vi "Begin.vi"(8 "error in":errorcluster) -> (0 "error out":errorcluster)   [LabVIEW 2016]
doc: "Called before other user functions, this VI is expected to open initial I/O refnums, load in file data, and do all program initialization. Notice that the <B>error out</B> terminal is simply used for data flow. Wiring it to other structures or subVIs ensures that this VI runs first."
uses:
  <vilib>/Rock Robotics/WPI/Solenoid/WPI_SolenoidValue.ctl
  <vilib>/Rock Robotics/WPI/ThirdParty/CanMotor/TalonSRX/WPI_CANTalonSRX_APIControlMode.ctl
  <vilib>/Rock Robotics/WPI/ThirdParty/CanMotor/TalonSRX/WPI_CANTalonSRX_BrakeOverride.ctl
  <vilib>/Rock Robotics/WPI/ThirdParty/CanMotor/TalonSRX/WPI_CANTalonSRX_APIFeedbackSelect.ctl
  <vilib>/Rock Robotics/WPI/SafetyOutput/WPI_SafetyOutputConfigMenu.ctl
  Constants/Private/Private Global.vi
  <vilib>/Rock Robotics/WPI/Solenoid/WPI_SolenoidOpenDouble.vi
  <vilib>/Rock Robotics/WPI/RobotDrive/WPI_RobotDriveOpen2MotorWithSPARK.vi
  <vilib>/Rock Robotics/WPI/MotorControl/WPI_MotorControlOpen SPARK.vi
  <vilib>/Rock Robotics/WPI/Counter/WPI_CounterDigitalInputToDigitalSource.vi
  <vilib>/Rock Robotics/Network Tables/NT Write String Array.vi
  <vilib>/Rock Robotics/WPI/Solenoid/WPI_SolenoidSetEnum.vi
  Constants/Constants.lvlib
  SubSystems/Path Track/Path Track.lvlib
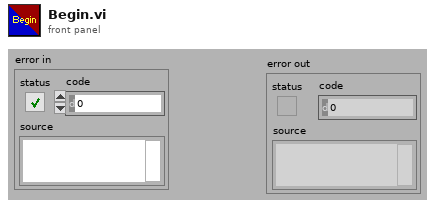
[diagram p1: front panel]
types:
  T1 = typedef "WPI_SafetyOutputConfigMenu.ctl" = enum16{"Enable", "Disable"}
  T2 = typedef "WPI_CANTalonSRX_APIControlMode.ctl" = enum8{"Percent VBus", "Speed", "Position", "Slave", "Unchanged / Invalid", "Voltage Compensation", "Current", "Motion Profile", "Motion Magic"}
  T3 = typedef "WPI_CANTalonSRX_APIFeedbackSelect.ctl" = enum16{"Digital Quadrature Encoder", "Analog Potentiometer", "Analog Encoder", "Count on Quad-A (Rising-Edge)", "Count on Quad-A (Falling-Edge)", "CTR Magnetic Enc (Absolute)", "CTR Magnetic Enc (Relative)", "Pulse Width"}
  T4 = typedef "WPI_CANTalonSRX_BrakeOverride.ctl" = enum8{"No Override", "Override to Coast", "Override to Brake"}
  T5 = typedef "WPI_SolenoidValue.ctl" = enum16{"Off", "On", "Forward", "Reverse"}
  T6 = typedef "Constants.lvlib/Constants.ctl" = cluster{"Port Layout":cluster{"RightMotorInverted":bool, "LeftMotorInverted":bool, "Left Motors":T7, "Right Motors":T7, "Auton List":string[], "XBOX Port":T8, "Encoder L A":T9, "Encoder L B":T9, "Encoder R A":T9, "Encoder R B":T9, "L Encoder Inverse":bool, "R Encoder Inverse":bool, "Drive Distance per Count":dbl, "Gyro Bus":T10, "Fuel Roller 1":T7, "Front Roller":T7, "Gear Flipper":T7, "Climber 1":T7, "Fuel Roller Invert":bool, "Front Roller Invert":bool, "Gear Flipper Invert":bool, "Climber Invert":bool, "PCM":u8, "Fuel Roller 2":T7, "Gear Sensor":T11, "Gear Release Fwd":T12, "Gear Release Rvrs":T12, "Fuel Arm Fwd":T12, "Fuel Arm Rvrs":T12, "Shifter Fwrd":T12, "Shifter Rvrs":T12, "Climber 2":T7, "PDP":u8, "Shooter Front Channel":u8, "Shooter Rear Channel":u8, "Shooter Feed Channel":u8, "Camera Servo":T7, "Gear Servo":T7, "Gear Puncher Fwrd":T12, "Gear Puncher Rvrs":T12, "Shooter Inverse":bool, "Ring Light Switch":T9}, "Drive Constants":cluster{"Wheelbase In.":dbl, "Max Velocity (In/sec)":dbl, "Max Accel (In/sec^2)":dbl, "Max Jerk (In/sec^3)":dbl, "Path dt":dbl, "Path Sample Count":i32, "Deadband":dbl}, "Arm System":cluster{"Front Roller Gear Speed":dbl, "Front Roller Fuel Speed":dbl, "Gear Flipper Speed":dbl, "Fuel Roller Speed":dbl, "Gear Release Wait (ms)":i32, "Gear Sensor Threshold":dbl, "Flappy Open Angle":i32, "Flappy Close Angle":i32, "Ramp Rate (EGU/min)":dbl}, "Shooter":cluster{"Shooter Wheels":cluster{"P":dbl, "I":dbl, "D":dbl, "F":dbl, "IZone":dbl}, "Feeder":cluster{"P":dbl, "I":dbl, "D":dbl, "F":dbl, "IZone":dbl}, "Front Shooter RPM":dbl, "Rear Shooter RPM":dbl, "Agitator Speed":dbl, "Feeder Speed":dbl, "Shooter CPR":u32, "Feeder CPR":u32}, "Vision":cluster{"High Goal Height (in.)":dbl, "Low Goal Height (in.)":dbl, "Camera Height High (in.)":dbl, "Camera Height Low (in.)":dbl, "Servo Pitch Gear (deg)":dbl, "Camera Yaw (deg)":dbl, "Servo Gear":i32, "Servo Boiler":i32, "Servo Pitch Boiler (deg)":dbl}}
  T7 = typedef "FPGA_DIOPWMChannel.ctl" = enum8{"PWM 0", "PWM 1", "PWM 2", "PWM 3", "PWM 4", "PWM 5", "PWM 6", "PWM 7", "PWM 8", "PWM 9", "PWM MXP 0", "PWM MXP 1", "PWM MXP 2", "PWM MXP 3", "PWM MXP 4", "PWM MXP 5", "PWM MXP 6", "PWM MXP 7", "PWM MXP 8", "PWM MXP 9", "Invalid"}
  T8 = typedef "WPI_JoystickDeviceEnum.ctl" = enum16{"USB 0", "USB 1", "USB 2", "USB 3", "USB 4", "USB 5"}
  T9 = typedef "FPGA_DIOChannel.ctl" = enum8{"DIO 0", "DIO 1", "DIO 2", "DIO 3", "DIO 4", "DIO 5", "DIO 6", "DIO 7", "DIO 8", "DIO 9", "DIO MXP 0", "DIO MXP 1", "DIO MXP 2", "DIO MXP 3", "DIO MXP 4", "DIO MXP 5", "DIO MXP 6", "DIO MXP 7", "DIO MXP 8", "DIO MXP 9", "DIO MXP 10", "DIO MXP 11", "DIO MXP 12", "DIO MXP 13", "DIO MXP 14", "DIO MXP 15", "SPI Port CS1", "SPI Port CS2", "SPI Port CS3", "SPI Port MISO", "SPI Port MOSI", "Invalid"}
  T10 = typedef "spi_bus.ctl" = enum16{"SPI On-Board, CS0", "SPI On-Board, CS1", "SPI On-Board, CS2", "SPI On-Board, CS3", "SPI MXP", "Invalid"}
  T11 = typedef "FPGA_AIChannel.ctl" = enum8{"AI 0", "AI 1", "AI 2", "AI 3", "AI MXP 0", "AI MXP 1", "AI MXP 2", "AI MXP 3", "Invalid"}
  T12 = typedef "WPI_SolenoidChannel.ctl" = enum8{"Solenoid 0", "Solenoid 1", "Solenoid 2", "Solenoid 3", "Solenoid 4", "Solenoid 5", "Solenoid 6", "Solenoid 7", "Invalid"}
  T13 = typedef "WPI_DigitalInputDevRef.ctl" = cluster{"DevStatus":errorcluster, "DIO Channel":T9}
  T14 = typedef "WPI_SolenoidDevRef.ctl" = cluster{"DevStatus":errorcluster, "Pneumatics Control Module":u8, "Forward Solenoid Channel":T12, "Reverse Solenoid Channel":T12}
  T15 = typedef "FPGA_CounterEncoderSourceConvertionLVSourceType.ctl" = cluster{"DevStatus":errorcluster, "AnalogTriggerMode?":bool, "DigitalMode":cluster{"DIO Channel":T16}, "AnalogTriggerMode":cluster{"AnalogTriggerIndex":T17, "OutputType":T18}}
  T16 = typedef "FPGA_DIODigitalSourceChannel.ctl" = enum8{"DIO 0", "DIO 1", "DIO 2", "DIO 3", "DIO 4", "DIO 5", "DIO 6", "DIO 7", "DIO 8", "DIO 9", "DIO MXP 0", "DIO MXP 1", "DIO MXP 2", "DIO MXP 3", "DIO MXP 4", "DIO MXP 5", "DIO MXP 6", "DIO MXP 7", "DIO MXP 8", "DIO MXP 9", "DIO MXP 10", "DIO MXP 11", "DIO MXP 12", "DIO MXP 13", "DIO MXP 14", "DIO MXP 15", "Disabled"}
  T17 = typedef "FPGA_AnalogTriggerIndex.ctl" = enum8{"Trig 0", "Trig 1", "Trig 2", "Trig 3", "Trig 4", "Trig 5", "Trig 6", "Trig 7", "Invalid"}
  T18 = typedef "FPGA_AnalogTriggerOutType.ctl" = enum16{"InWindow", "TriggerState", "Rising", "Falling"}
  T19 = typedef "WPI_JoystickDevRef.ctl" = cluster{"Device":T8}
  T20 = typedef "WPI_RobotDriveDevRef.ctl" = cluster{"DevStatus":errorcluster, "Motors[]":T21[], "Square Inputs":bool, "Max Output":dbl}
  T21 = typedef "WPI_MotorControlDeviceRef.ctl" = cluster{"DeviceStatus":errorcluster, "Type":T22, "PWM":cluster{"PWM Channel":T7, "DeadBand":T23}, "CAN":cluster{"Device Number":u8, "SetOutput VI Ref":variant, "GetOutput VI Ref":variant, "Enable VI Ref":variant, "Disable VI Ref":variant, "Data":variant}, "Invert":bool}
  T22 = typedef "WPI_MotorControlType.ctl" = enum16{"PWM", "CAN"}
  T23 = typedef "WPI_PWMDeadband.ctl" = cluster{"Name":string, "maxPositivePwm":i32, "minPositivePwm":i32, "centerPwm":i32, "maxNegativePwm":i32, "minNegativePwm":i32, "angularRange":u16}
  T24 = typedef "WPI_EncoderDevRef.ctl" = cluster{"DevStatus":errorcluster, "EncoderIndex":T25, "CounterIndex":T26, "DistancePerCount":dbl, "Decoding Type":T27}
  T25 = typedef "FPGA_EncoderIdx.ctl" = enum8{"Enc 0", "Enc 1", "Enc 2", "Enc 3", "Enc 4", "Enc 5", "Enc 6", "Enc 7", "Invalid"}
  T26 = typedef "FPGA_CounterCtrSystemIndex.ctl" = enum8{"Ctr 0", "Ctr 1", "Ctr 2", "Ctr 3", "Ctr 4", "Ctr 5", "Ctr 6", "Ctr 7", "Invalid"}
  T27 = typedef "WPI_EncoderType.ctl" = enum16{"1x", "2x", "4x"}
  T28 = typedef "WPI_DigitalOutputDevRef.ctl" = cluster{"DIO Channel":T9, "DevStatus":errorcluster}
  T29 = typedef "WPI_ServoDeviceRef.ctl" = cluster{"DeviceStatus":errorcluster, "PWM Channel":T7, "DeadBand":T23}
  T30 = typedef "WPI_AnalogChannelDevRef.ctl" = cluster{"DevStatus":errorcluster, "Analog Channel":T11}
  T31 = typedef "WPI_GyroDevRef.ctl" = cluster{"DevStatus":errorcluster, "Analog Channel":T11, "Offset":dbl, "Gain (VoltsPerDegree/Second)":dbl, "Gyro Type":enum16{"Analog", "XRS450"}, "Handle":i32, "SPI Bus":T10, "Device Found":bool, "Sample Rate":dbl, "Calibrate On Open":bool}
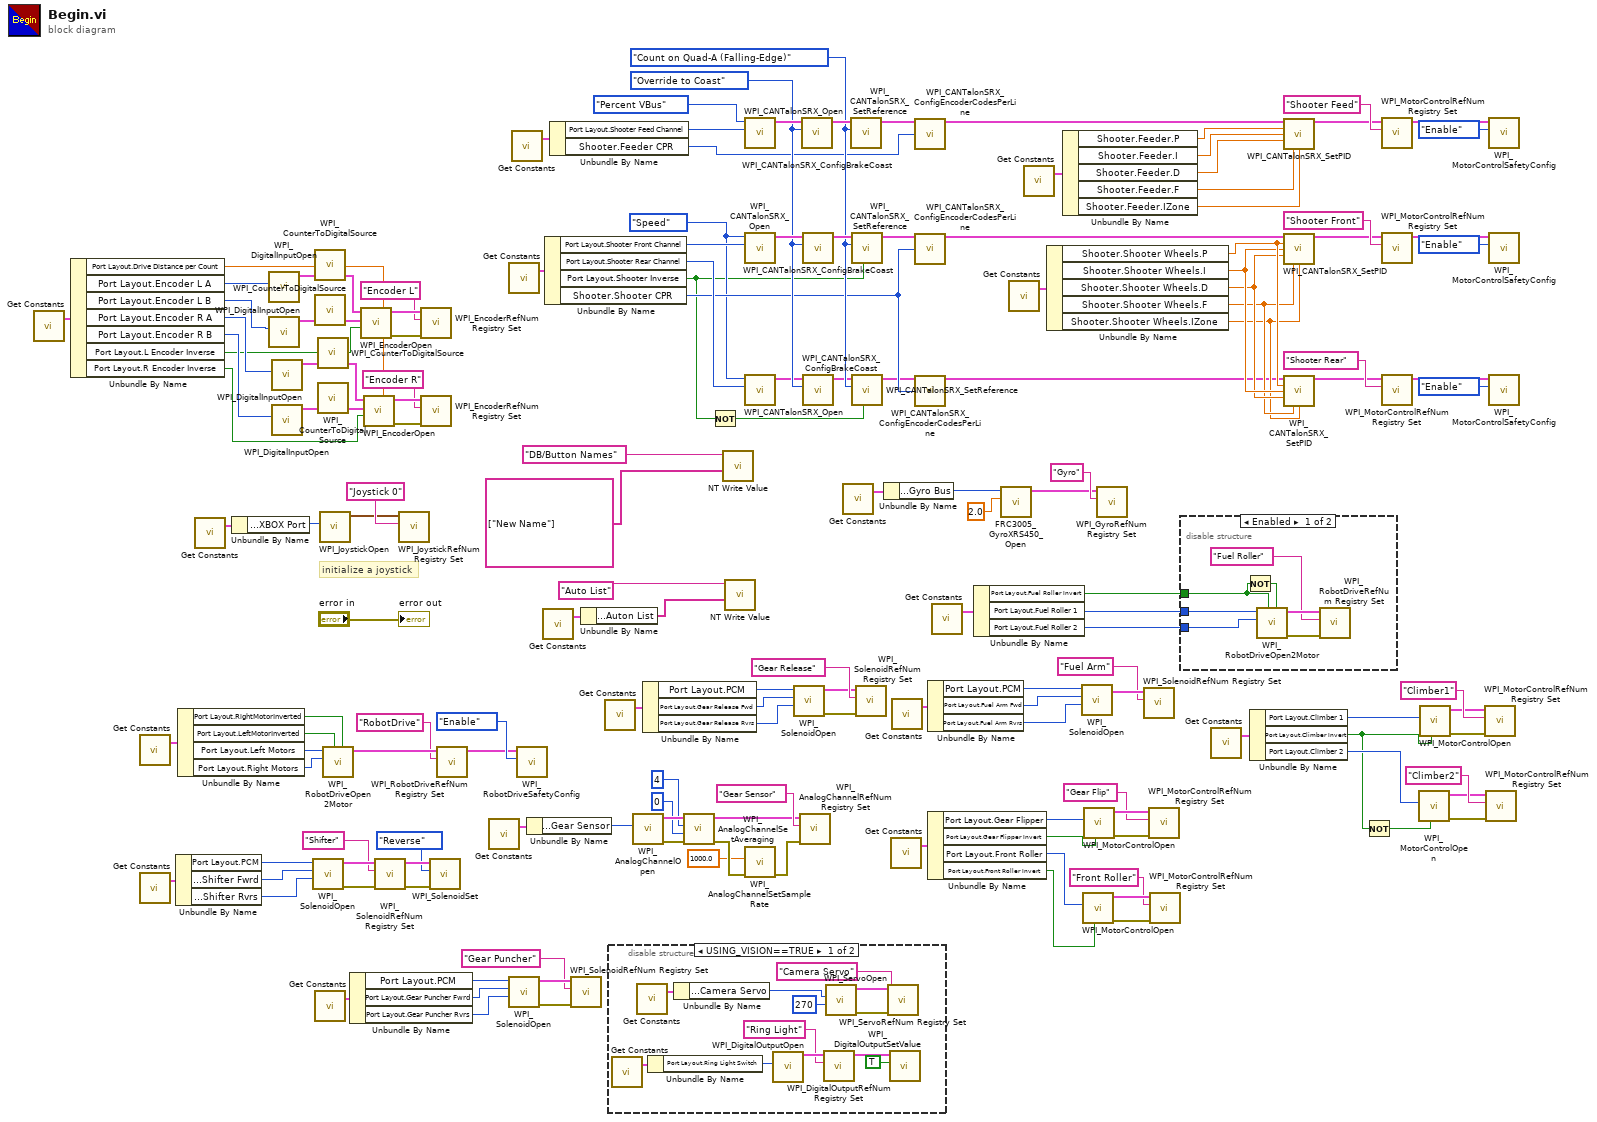
[diagram p0: block diagram]
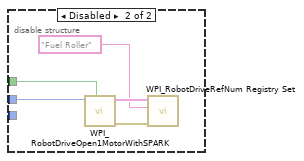
[diagram p3: hidden frame]
diagram:
  w3 = WPI_CANTalonSRX_APIControlMode."Speed" ("Control Mode")
  w29 = WPI_CANTalonSRX_APIFeedbackSelect."Count on Quad-A (Falling-Edge)" ("Feedback Reference")
  w32 = WPI_CANTalonSRX_BrakeOverride."Override to Coast" ("Brake / Coast Mode")
  # "initialize a joystick"
  n1 = call "Get Constants.vi"() -> ("Constants"=w72:T6)  [unwired: 3 in]
  n2 = Unbundle By Name(w72) -> ("Port Layout.Drive Distance per Count"=w130:dbl, "Port Layout.Encoder L A"=w144:T9, "Port Layout.Encoder L B"=w143:T9, "Port Layout.Encoder R A"=w142:T9, "Port Layout.Encoder R B"=w141:T9, "Port Layout.L Encoder Inverse"=w140:bool, "Port Layout.R Encoder Inverse"=w139:bool)
  n3 = call "Get Constants.vi"() -> ("Constants"=w86:T6)  [unwired: 3 in]
  n4 = call "Get Constants.vi"() -> ("Constants"=w77:T6)  [unwired: 3 in]
  n5 = Unbundle By Name(w77) -> ("Port Layout.PCM"=w78:u8, "Port Layout.Shifter Fwrd"=w81:T12, "Port Layout.Shifter Rvrs"=w80:T12)
  n6 = Unbundle By Name(w86) -> ("Port Layout.RightMotorInverted"=w82:bool, "Port Layout.LeftMotorInverted"=w83:bool, "Port Layout.Left Motors"=w84:T7, "Port Layout.Right Motors"=w85:T7)
  n7 = call "Get Constants.vi"() -> ("Constants"=w156:T6)  [unwired: 3 in]
  n8 = Unbundle By Name(w156) -> ("Port Layout.XBOX Port"=w155:T8)
  n9 = call <vilib>:"WPI_DigitalInputOpen.vi"("DIO Channel"=w144) -> ("DigitalInputDevRef"=w151:T13)  [unwired: 1 in, 9 out]
  n10 = call <vilib>:"WPI_DigitalInputOpen.vi"("DIO Channel"=w143) -> ("DigitalInputDevRef"=w150:T13)  [unwired: 1 in, 9 out]
  n11 = call <vilib>:"WPI_DigitalInputOpen.vi"("DIO Channel"=w142) -> ("DigitalInputDevRef"=w146:T13)  [unwired: 1 in, 9 out]
  n12 = call <vilib>:"WPI_DigitalInputOpen.vi"("DIO Channel"=w141) -> ("DigitalInputDevRef"=w147:T13)  [unwired: 1 in, 9 out]
  n13 = call-poly <vilib>:"WPI_SolenoidOpen.vi"("Reverse Solenoid Channel"=w80, "Forward Solenoid Channel"=w81, "Pneumatics Control Module (0)"=w78) -> ("error out"=w79:errorcluster, "SolenoidDevRef"=w76:T14)  [unwired: 7 in]
  n14 = call-poly <vilib>:"WPI_CounterToDigitalSource.vi"("DigitalInputDevRef"=w151) -> ("Digital Source"=w152:T15)  [unwired: 6 out]
  n15 = call-poly <vilib>:"WPI_CounterToDigitalSource.vi"("DigitalInputDevRef"=w150) -> ("Digital Source"=w149:T15)  [unwired: 6 out]
  n16 = call "Get Constants.vi"() -> ("Constants"=w56:T6)  [unwired: 3 in]
  n17 = call-poly <vilib>:"WPI_CounterToDigitalSource.vi"("DigitalInputDevRef"=w146) -> ("Digital Source"=w145:T15)  [unwired: 6 out]
  n18 = call-poly <vilib>:"WPI_CounterToDigitalSource.vi"("DigitalInputDevRef"=w147) -> ("Digital Source"=w148:T15)  [unwired: 6 out]
  n19 = call <vilib>:"WPI_JoystickOpen.vi"("JoystickDevice"=w155) -> ("JoystickDevRef"=w161:T19)  [unwired: 10 in]
  n20 = call-poly <vilib>:"WPI_RobotDriveOpen2Motor.vi"("Right Motor Inverted"=w82, "Left Motor Inverted"=w83, "Right Motor"=w85, "Left Motor"=w84) -> ("RobotDriveDevRef"=w89:T20)  [unwired: 6 in, 1 out]
  n21 = Unbundle By Name(w56) -> ("Port Layout.PCM"=w57:u8, "Port Layout.Gear Puncher Fwrd"=w60:T12, "Port Layout.Gear Puncher Rvrs"=w59:T12)
  n22 = call <vilib>:"WPI_EncoderOpen.vi"("DistancePerCount"=w130, "Invert Direction (False)"=w140, "BSource"=w149, "ASource"=w152) -> ("error out"=w138:errorcluster, "EncoderDevRef"=w137:T24)  [unwired: 4 in, 2 out]
  n23 = call <vilib>:"WPI_EncoderOpen.vi"("DistancePerCount"=w130, "Invert Direction (False)"=w139, "BSource"=w148, "ASource"=w145) -> ("error out"=w136:errorcluster, "EncoderDevRef"=w135:T24)  [unwired: 4 in, 2 out]
  n24 = call <vilib>:"WPI_SolenoidRefNum Registry Set.vi"("error in (no error)"=w79, "refnum name"="Shifter", "SolenoidDevRef"=w76) -> ("error out"=w53:errorcluster, "SolenoidDevRef"=w52:T14)  [unwired: 7 in]
  n25 = call <vilib>:"WPI_JoystickRefNum Registry Set.vi"("refnum name"="Joystick 0", "JoystickDevRef"=w161) -> ()  [unwired: 8 in, 2 out]
  n26 = call <vilib>:"WPI_EncoderRefNum Registry Set.vi"("error in (no error)"=w138, "refnum name"="Encoder L", "EncoderDevRef"=w137) -> ()  [unwired: 7 in, 2 out]
  n27 = call <vilib>:"WPI_EncoderRefNum Registry Set.vi"("error in (no error)"=w136, "refnum name"="Encoder R", "EncoderDevRef"=w135) -> ()  [unwired: 7 in, 2 out]
  n28 = call-poly <vilib>:"WPI_SolenoidSet.vi"("error in (no error)"=w53, "Value"=WPI_SolenoidValue."Reverse", "SolenoidDevRef"=w52) -> ()  [unwired: 7 in, 2 out]
  n29 = call <vilib>:"WPI_RobotDriveRefNum Registry Set.vi"("refnum name"="RobotDrive", "RobotDriveDevRef"=w89) -> ("RobotDriveDevRef"=w88:T20)  [unwired: 8 in, 1 out]
  n30 = call "Get Constants.vi"() -> ("Constants"=w105:T6)  [unwired: 3 in]
  n31 = call "Get Constants.vi"() -> ("Constants"=w45:T6)  [unwired: 3 in]
  n32 = call-poly <vilib>:"WPI_SolenoidOpen.vi"("Reverse Solenoid Channel"=w59, "Forward Solenoid Channel"=w60, "Pneumatics Control Module (0)"=w57) -> ("error out"=w58:errorcluster, "SolenoidDevRef"=w55:T14)  [unwired: 7 in]
  n33 = call "Get Constants.vi"() -> ("Constants"=w42:T6)  [unwired: 3 in]
  n34 = call <vilib>:"WPI_RobotDriveSafetyConfig.vi"("mode"=WPI_SafetyOutputConfigMenu."Enable", "RobotDriveDevRef"=w88) -> ()  [unwired: 8 in, 2 out]
  n35 = Unbundle By Name(w105) -> ("Port Layout.Gear Sensor"=w100:T11)
  n36 = call "Get Constants.vi"() -> ("Constants"=w154:T6)  [unwired: 3 in]
  n37 = Unbundle By Name(w45) -> ("Port Layout.Shooter Front Channel"=w44:u8, "Port Layout.Shooter Rear Channel"=w43:u8, "Port Layout.Shooter Inverse"=w1:bool, "Shooter.Shooter CPR"=w12:u32)
  n38 = Unbundle By Name(w42) -> ("Port Layout.Shooter Feed Channel"=w37:u8, "Shooter.Feeder CPR"=w14:u32)
  n39 = call <vilib>:"WPI_SolenoidRefNum Registry Set.vi"("error in (no error)"=w58, "refnum name"="Gear Puncher", "SolenoidDevRef"=w55) -> ()  [unwired: 7 in, 2 out]
  n40 = Unbundle By Name(w154) -> ("Port Layout.Auton List"=w153:string[])
  n41 = call "Get Constants.vi"() -> ("Constants"=w108:T6)  [unwired: 3 in]
  n42 = disable-structure shown="USING_VISION==TRUE" {
    frame condition #0 (active) {
      n43 = call "Get Constants.vi"() -> ("Constants"=w168:T6)  [unwired: 3 in]
      n44 = call "Get Constants.vi"() -> ("Constants"=w173:T6)  [unwired: 3 in]
      n45 = Unbundle By Name(w168) -> ("Port Layout.Ring Light Switch"=w167:T9)
      n46 = Unbundle By Name(w173) -> ("Port Layout.Camera Servo"=w174:T7)
      n47 = call <vilib>:"WPI_DigitalOutputOpen.vi"("DIO Channel"=w167) -> ("DigitalOutputDevRef"=w166:T28)  [unwired: 9 in, 1 out]
      n48 = call <vilib>:"WPI_DigitalOutputRefNum Registry Set.vi"("refnum name"="Ring Light", "DigitalOutputDevRef"=w166) -> ("DigitalOutputDevRef"=w164:T28)  [unwired: 8 in, 1 out]
      n49 = call <vilib>:"WPI_ServoOpen.vi"("Angular Range"=u16 270, "PWM Channel"=w174) -> ("error out"=w169:errorcluster, "ServoDeviceRef"=w170:T29)  [unwired: 8 in]
      n50 = call <vilib>:"WPI_ServoRefNum Registry Set.vi"("error in (no error)"=w169, "refnum name"="Camera Servo", "ServoDeviceRef"=w170) -> ()  [unwired: 7 in, 2 out]
      n51 = call <vilib>:"WPI_DigitalOutputSetValue.vi"("Value"=TRUE, "DigitalOutputDevRef"=w164) -> ()  [unwired: 8 in, 2 out]
    }
    frame condition #1 {
    }
  }
  n52 = call <vilib>:"WPI_AnalogChannelOpen.vi"("Analog Channel"=w100) -> ("error out"=w99:errorcluster, "AIDeviceRef"=w97:T30)  [unwired: 2 in, 7 out]
  n53 = Unbundle By Name(w108) -> ("Port Layout.PCM"=w107:u8, "Port Layout.Gear Release Fwd"=w101:T12, "Port Layout.Gear Release Rvrs"=w102:T12)
  n54 = call <vilib>:"WPI_AnalogChannelSetAveraging.vi"("error in (no error)"=w99, "OversampleBits"=u8 0, "AverageBits"=u8 4, "AIDeviceRef"=w97) -> ("error out"=w98:errorcluster, "AIDeviceRef"=w94:T30)  [unwired: 6 in]
  n55 = Not(x=w1) -> (.not. x?=w2:bool)
  n56 = call-poly <vilib>:"NT Write Value.vi"("String Array"=string[] ["New Name"], "Name"="DB/Button Names") -> ()  [unwired: 9 in, 1 out]
  n57 = call-poly <vilib>:"NT Write Value.vi"("String Array"=w153, "Name"="Auto List") -> ()  [unwired: 9 in, 1 out]
  n58 = call <vilib>:"WPI_CANTalonSRX_Open.vi"("Device Number"=w37, "Control Mode"=WPI_CANTalonSRX_APIControlMode."Percent VBus") -> ("CAN Talon SRX Ref"=w41:T21)  [unwired: 8 in, 1 out]
  n59 = call <vilib>:"WPI_CANTalonSRX_Open.vi"("Device Number"=w44, "Control Mode"=w3) -> ("CAN Talon SRX Ref"=w46:T21)  [unwired: 8 in, 1 out]
  n60 = call <vilib>:"WPI_CANTalonSRX_Open.vi"("Device Number"=w43, "Control Mode"=w3) -> ("CAN Talon SRX Ref"=w11:T21)  [unwired: 8 in, 1 out]
  n61 = call <vilib>:"WPI_AnalogChannelSetSampleRate.vi"("error in (no error)"=w98, "Samples Per Second (per channel)"=1000.0) -> ("error out"=w95:errorcluster)  [unwired: 9 in]
  n62 = call-poly <vilib>:"WPI_SolenoidOpen.vi"("Reverse Solenoid Channel"=w102, "Forward Solenoid Channel"=w101, "Pneumatics Control Module (0)"=w107) -> ("error out"=w106:errorcluster, "SolenoidDevRef"=w109:T14)  [unwired: 7 in]
  n63 = call <vilib>:"WPI_AnalogChannelRefNum Registry Set.vi"("error in (no error)"=w95, "refnum name"="Gear Sensor", "AIDeviceRef"=w94) -> ()  [unwired: 7 in, 2 out]
  n64 = call <vilib>:"WPI_CANTalonSRX_ConfigBrakeCoast.vi"("Brake / Coast Mode"=w32, "CAN Talon SRX Ref"=w41) -> ("CAN Talon SRX Ref"=w34:T21)  [unwired: 8 in, 1 out]
  n65 = call <vilib>:"WPI_CANTalonSRX_ConfigBrakeCoast.vi"("Brake / Coast Mode"=w32, "CAN Talon SRX Ref"=w46) -> ("CAN Talon SRX Ref"=w33:T21)  [unwired: 8 in, 1 out]
  n66 = call <vilib>:"WPI_CANTalonSRX_ConfigBrakeCoast.vi"("Brake / Coast Mode"=w32, "CAN Talon SRX Ref"=w11) -> ("CAN Talon SRX Ref"=w6:T21)  [unwired: 8 in, 1 out]
  n67 = call "Get Constants.vi"() -> ("Constants"=w74:T6)  [unwired: 3 in]
  n68 = call <vilib>:"WPI_CANTalonSRX_SetReference.vi"("Feedback Reference"=w29, "CAN Talon SRX Ref"=w34) -> ("CAN Talon SRX Ref"=w30:T21)  [unwired: 8 in, 1 out]
  n69 = call <vilib>:"WPI_CANTalonSRX_SetReference.vi"("Reverse Closed-Loop Output"=w1, "Feedback Reference"=w29, "CAN Talon SRX Ref"=w33) -> ("CAN Talon SRX Ref"=w31:T21)  [unwired: 7 in, 1 out]
  n70 = call <vilib>:"WPI_CANTalonSRX_SetReference.vi"("Reverse Closed-Loop Output"=w2, "Feedback Reference"=w29, "CAN Talon SRX Ref"=w6) -> ("CAN Talon SRX Ref"=w5:T21)  [unwired: 7 in, 1 out]
  n71 = call <vilib>:"WPI_SolenoidRefNum Registry Set.vi"("error in (no error)"=w106, "refnum name"="Gear Release", "SolenoidDevRef"=w109) -> ()  [unwired: 7 in, 2 out]
  n72 = Unbundle By Name(w74) -> ("Port Layout.Gyro Bus"=w73:T10)
  n73 = call "Get Constants.vi"() -> ("Constants"=w115:T6)  [unwired: 3 in]
  n74 = call "Get Constants.vi"() -> ("Constants"=w124:T6)  [unwired: 3 in]
  n75 = call <vilib>:"WPI_CANTalonSRX_ConfigEncoderCodesPerLine.vi"("CAN Talon SRX Ref"=w30, "Number Encoder Lines\n(Counts Per Rotation)"=w14) -> ("CAN Talon SRX Ref"=w16:T21)  [unwired: 12 in, 1 out]
  n76 = call <vilib>:"WPI_CANTalonSRX_ConfigEncoderCodesPerLine.vi"("CAN Talon SRX Ref"=w31, "Number Encoder Lines\n(Counts Per Rotation)"=w12) -> ("CAN Talon SRX Ref"=w15:T21)  [unwired: 12 in, 1 out]
  n77 = call <vilib>:"WPI_CANTalonSRX_ConfigEncoderCodesPerLine.vi"("CAN Talon SRX Ref"=w5, "Number Encoder Lines\n(Counts Per Rotation)"=w12) -> ("CAN Talon SRX Ref"=w4:T21)  [unwired: 12 in, 1 out]
  n78 = Unbundle By Name(w124) -> ("Port Layout.PCM"=w125:u8, "Port Layout.Fuel Arm Fwd"=w103:T12, "Port Layout.Fuel Arm Rvrs"=w104:T12)
  n79 = Unbundle By Name(w115) -> ("Port Layout.Gear Flipper"=w112:T7, "Port Layout.Gear Flipper Invert"=w111:bool, "Port Layout.Front Roller"=w114:T7, "Port Layout.Front Roller Invert"=w113:bool)
  n80 = call "Get Constants.vi"() -> ("Constants"=w123:T6)  [unwired: 3 in]
  n81 = Unbundle By Name(w123) -> ("Port Layout.Fuel Roller Invert"=w120:bool, "Port Layout.Fuel Roller 1"=w122:T7, "Port Layout.Fuel Roller 2"=w121:T7)
  n82 = call "FRC3005_GyroXRS450_Open.vi"("Sample Rate (ms)"=2.0, "SPI Bus"=w73) -> ("GyroDeviceRef"=w131:T31)  [unwired: 8 in, 1 out]
  n83 = call "Get Constants.vi"() -> ("Constants"=w28:T6)  [unwired: 3 in]
  n84 = call "Get Constants.vi"() -> ("Constants"=w27:T6)  [unwired: 3 in]
  n85 = Unbundle By Name(w28) -> ("Shooter.Shooter Wheels.P"=w21:dbl, "Shooter.Shooter Wheels.I"=w20:dbl, "Shooter.Shooter Wheels.D"=w19:dbl, "Shooter.Shooter Wheels.F"=w18:dbl, "Shooter.Shooter Wheels.IZone"=w17:dbl)
  n86 = Unbundle By Name(w27) -> ("Shooter.Feeder.P"=w25:dbl, "Shooter.Feeder.I"=w26:dbl, "Shooter.Feeder.D"=w24:dbl, "Shooter.Feeder.F"=w23:dbl, "Shooter.Feeder.IZone"=w22:dbl)
  n87 = call-poly <vilib>:"WPI_SolenoidOpen.vi"("Reverse Solenoid Channel"=w104, "Forward Solenoid Channel"=w103, "Pneumatics Control Module (0)"=w125) -> ("SolenoidDevRef"=w119:T14)  [unwired: 7 in, 1 out]
  n88 = call-poly <vilib>:"WPI_MotorControlOpen.vi"("Invert"=w113, "PWM Channel"=w114) -> ("error out"=w116:errorcluster, "MotorControlDeviceRef"=w129:T21)  [unwired: 8 in]
  n89 = call-poly <vilib>:"WPI_MotorControlOpen.vi"("Invert"=w111, "PWM Channel"=w112) -> ("error out"=w117:errorcluster, "MotorControlDeviceRef"=w128:T21)  [unwired: 8 in]
  n90 = call <vilib>:"WPI_GyroRefNum Registry Set.vi"("refnum name"="Gyro", "GyroDevRef"=w131) -> ()  [unwired: 8 in, 2 out]
  n91 = call <vilib>:"WPI_SolenoidRefNum Registry Set.vi"("refnum name"="Fuel Arm", "SolenoidDevRef"=w119) -> ()  [unwired: 8 in, 2 out]
  n92 = call <vilib>:"WPI_MotorControlRefNum Registry Set.vi"("error in (no error)"=w117, "refnum name"="Gear Flip", "MotorControlDevRef"=w128) -> ()  [unwired: 7 in, 2 out]
  n93 = call <vilib>:"WPI_MotorControlRefNum Registry Set.vi"("error in (no error)"=w116, "refnum name"="Front Roller", "MotorControlDevRef"=w129) -> ()  [unwired: 7 in, 2 out]
  n94 = disable-structure shown="Enabled" {
    disable-tunnel: w122 -> [w181 w186]
    disable-tunnel: w121 -> [w180 _]
    disable-tunnel: w120 -> [w179 w185]
    frame Enabled {
      n95 = Not(x=w179) -> (.not. x?=w178:bool)
      n96 = call-poly <vilib>:"WPI_RobotDriveOpen2Motor.vi"("Right Motor Inverted"=w178, "Left Motor Inverted"=w179, "Right Motor"=w180, "Left Motor"=w181) -> ("error out"=w175:errorcluster, "RobotDriveDevRef"=w177:T20)  [unwired: 6 in]
      n97 = call <vilib>:"WPI_RobotDriveRefNum Registry Set.vi"("error in (no error)"=w175, "refnum name"="Fuel Roller", "RobotDriveDevRef"=w177) -> ()  [unwired: 7 in, 2 out]
    }
    frame Disabled {
      n98 = call <vilib>:"WPI_RobotDriveOpen1MotorWithSPARK.vi"("Motor Inverted"=w185, "Motor"=w186) -> ("error out"=w182:errorcluster, "RobotDriveDevRef"=w184:T20)  [unwired: 8 in]
      n99 = call <vilib>:"WPI_RobotDriveRefNum Registry Set.vi"("error in (no error)"=w182, "refnum name"="Fuel Roller", "RobotDriveDevRef"=w184) -> ()  [unwired: 7 in, 2 out]
    }
  }
  n100 = call "Get Constants.vi"() -> ("Constants"=w69:T6)  [unwired: 3 in]
  n101 = Unbundle By Name(w69) -> ("Port Layout.Climber 1"=w71:T7, "Port Layout.Climber Invert"=w61:bool, "Port Layout.Climber 2"=w70:T7)
  n102 = call <vilib>:"WPI_CANTalonSRX_SetPID.vi"("CAN Talon SRX Ref"=w16, "P"=w25, "I"=w26, "D"=w24, "F"=w23, "I Zone"=w22) -> ("CAN Talon SRX Ref"=w36:T21)  [unwired: 8 in, 1 out]
  n103 = call <vilib>:"WPI_CANTalonSRX_SetPID.vi"("CAN Talon SRX Ref"=w15, "P"=w21, "I"=w20, "D"=w19, "F"=w18, "I Zone"=w17) -> ("CAN Talon SRX Ref"=w35:T21)  [unwired: 8 in, 1 out]
  n104 = call <vilib>:"WPI_CANTalonSRX_SetPID.vi"("CAN Talon SRX Ref"=w4, "P"=w21, "I"=w20, "D"=w19, "F"=w18, "I Zone"=w17) -> ("CAN Talon SRX Ref"=w7:T21)  [unwired: 8 in, 1 out]
  n105 = Not(x=w61) -> (.not. x?=w62:bool)
  n106 = call <vilib>:"WPI_MotorControlRefNum Registry Set.vi"("refnum name"="Shooter Feed", "MotorControlDevRef"=w36) -> ("MotorControlDevRef"=w39:T21)  [unwired: 8 in, 1 out]
  n107 = call <vilib>:"WPI_MotorControlRefNum Registry Set.vi"("refnum name"="Shooter Front", "MotorControlDevRef"=w35) -> ("MotorControlDevRef"=w48:T21)  [unwired: 8 in, 1 out]
  n108 = call <vilib>:"WPI_MotorControlRefNum Registry Set.vi"("refnum name"="Shooter Rear", "MotorControlDevRef"=w7) -> ("MotorControlDevRef"=w9:T21)  [unwired: 8 in, 1 out]
  n109 = call-poly <vilib>:"WPI_MotorControlOpen.vi"("Invert"=w62, "PWM Channel"=w70) -> ("error out"=w68:errorcluster, "MotorControlDeviceRef"=w63:T21)  [unwired: 8 in]
  n110 = call-poly <vilib>:"WPI_MotorControlOpen.vi"("Invert"=w61, "PWM Channel"=w71) -> ("error out"=w67:errorcluster, "MotorControlDeviceRef"=w64:T21)  [unwired: 8 in]
  n111 = call <vilib>:"WPI_MotorControlRefNum Registry Set.vi"("error in (no error)"=w67, "refnum name"="Climber1", "MotorControlDevRef"=w64) -> ()  [unwired: 7 in, 2 out]
  n112 = call <vilib>:"WPI_MotorControlRefNum Registry Set.vi"("error in (no error)"=w68, "refnum name"="Climber2", "MotorControlDevRef"=w63) -> ()  [unwired: 7 in, 2 out]
  n113 = call <vilib>:"WPI_MotorControlSafetyConfig.vi"("mode"=WPI_SafetyOutputConfigMenu."Enable", "MotorControlDevRef"=w39) -> ()  [unwired: 8 in, 2 out]
  n114 = call <vilib>:"WPI_MotorControlSafetyConfig.vi"("mode"=WPI_SafetyOutputConfigMenu."Enable", "MotorControlDevRef"=w48) -> ()  [unwired: 8 in, 2 out]
  n115 = call <vilib>:"WPI_MotorControlSafetyConfig.vi"("mode"=WPI_SafetyOutputConfigMenu."Enable", "MotorControlDevRef"=w9) -> ()  [unwired: 8 in, 2 out]
  "error out" <- "error in"
